vi "Stop Trigger Example.vi"() -> ()   [LabVIEW 2021]
uses:
  <vilib>/DAQmx/configure/timing.llb/DAQmx Timing (Sample Clock).vi
  <vilib>/DAQmx/configure/trigger.llb/DAQmx Reference Trigger (Digital Edge).vi
  <vilib>/DAQmx/create/channels.llb/DAQmx Create Channel (AI-Voltage-Basic).vi
  <vilib>/Utility/error.llb/DialogType.ctl
  <resource>/objmgr/daqmx.rc
  <vilib>/DAQmx/read.llb/DAQmx Read (Analog 1D Wfm NChan NSamp).vi
  <vilib>/DAQmx/configure/trigger.llb/DAQmx Start Trigger (Digital Edge).vi
panel:
  in  "Physical Channel(s)":tag="Dev1/ai0" caption="Physical Channel"
  in  "Sample Rate 2":dbl=10000.0 caption="Rate (Hz)" format="%0.2f"
  in  "Minimum Value":dbl=-10.0 format="%0.2f"
  in  "Maximum Value":dbl=10.0 format="%0.2f"
  in  "Stop Trigger Source":tag="/Dev1/PFI0"
  in  "Buffer Size 2":u32=100000
  out "data":waveform(dbl)[](array[waveform])
  in  "Start Trigger Source":tag="/Dev1/PFI1"
  in  "Post-Trigger Samples":u32
  in  "Samples Per Read":u32=100
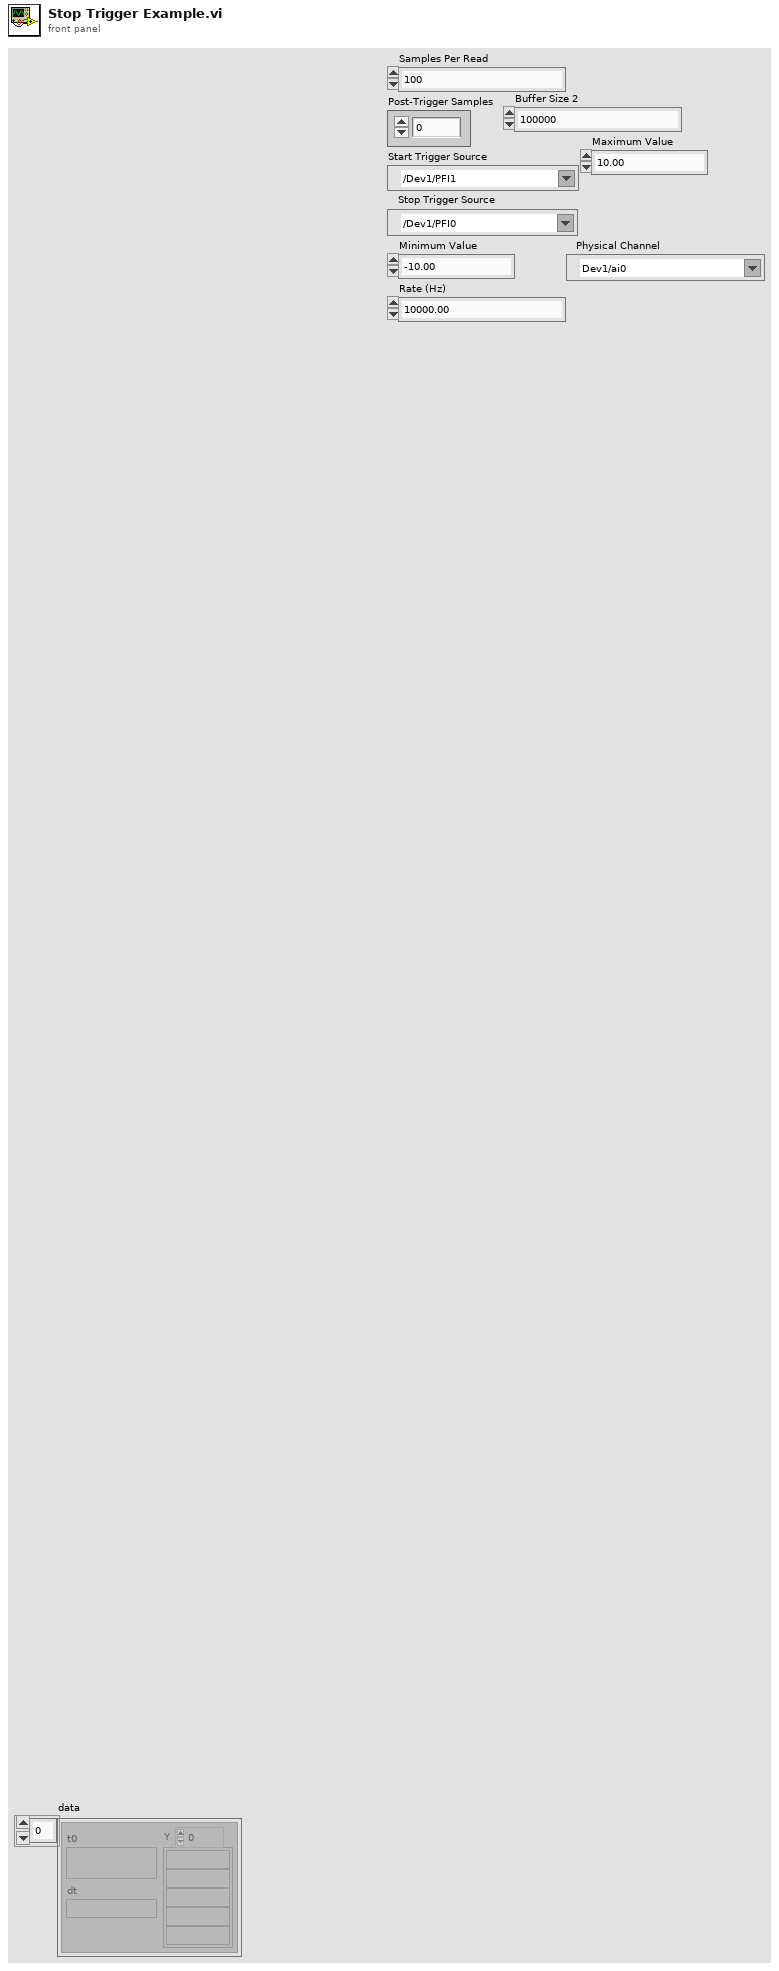
[diagram p1: front panel]
types:
  T1 = typedef "DialogType.ctl" = u16
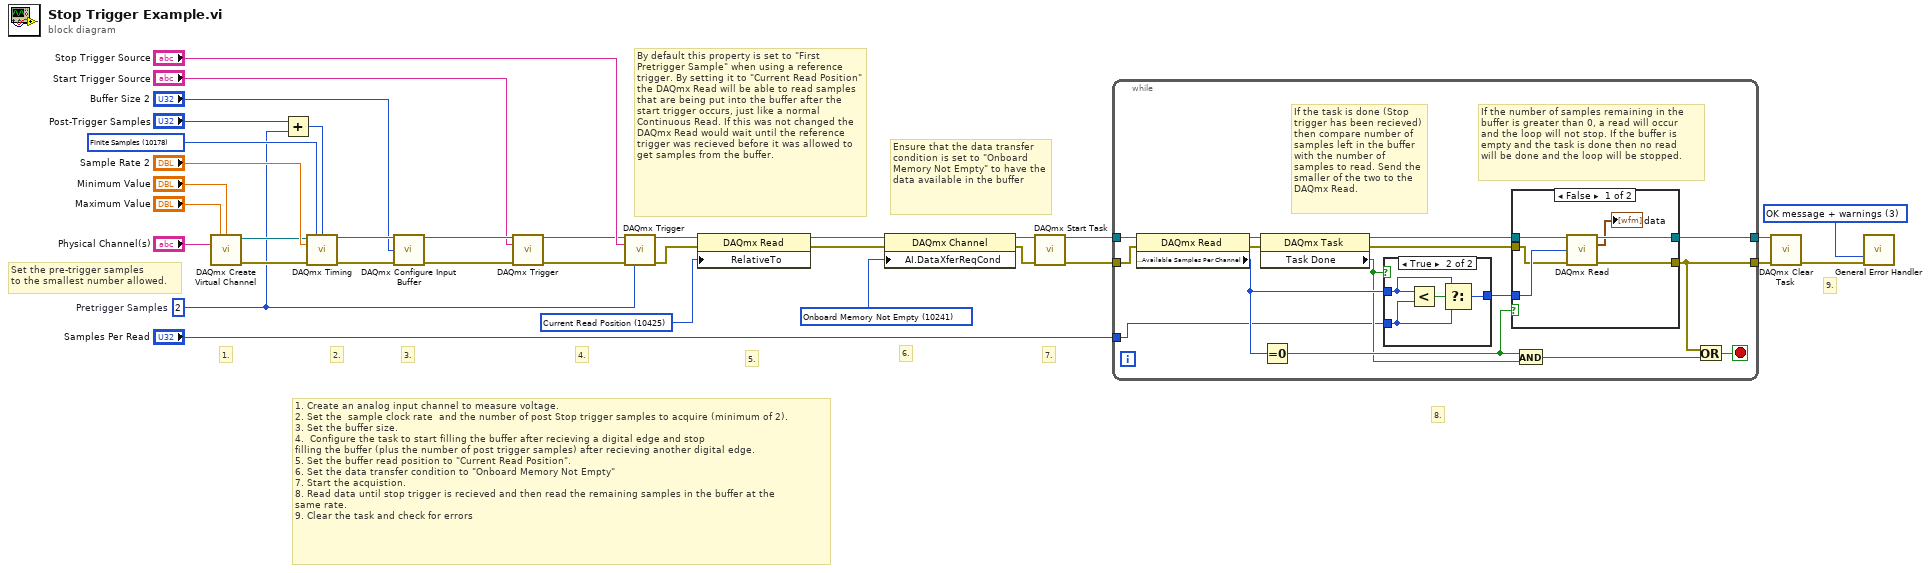
[diagram p0: block diagram]
diagram:
  w3 = 10241 items=["Onboard Memory More than Half Full"=10237, "Onboard Memory Not Empty"=10241, "Onboard Memory Custom Threshold"=12577, "When Acquisition Complete"=12546] ("AI.DataXferReqCond")
  w18 = 10425 items=["First Sample"=10424, "Current Read Position"=10425, "Reference Trigger"=10426, "First Pretrigger Sample"=10427, "Most Recent Sample"=10428] ("RelativeTo")
  w8 = u32 2  # Pretrigger Samples
  w24 = T1 3 items=["no dialog", "OK message", "continue or stop message", "OK message + warnings", "continue/stop + warnings"] ("type of dialog (OK msg:1)")
  w26 = 10178 items=["Finite Samples"=10178, "Continuous Samples"=10123] ("sample mode")
  # "Ensure that the data transfer condition is set to \"Onboard Memory Not Empty\" to have the data available in the buffer"
  # "7."
  # "Set the pre-trigger samples\nto the smallest number allowed."
  # "9."
  # "8."
  # "6."
  # "By default this property is set to \"First Pretrigger Sample\" when using a reference trigger. By setting it to \"Current Read Position\" the DAQmx Read will be able to read samples that are being put into the buffer after the start trigger occurs, just like a normal Continuous Read. If this was not changed the DAQmx Read would wait until the reference trigger was recieved before it was allowed to get samples from the buffer."
  # "5."
  # "1. Create an analog input channel to measure voltage.\n2. Set the  sample clock rate  and the number of post Stop trigger samples to acquire (minimum of 2).\n3. Set the buffer size.\n4.  Configure the task to start filling the buffer after recieving a digital edge and stop \nfilling the buffer (plus the number of post trigger samples) after recieving another digital edge.\n5. Set the buffer read position to \"Current Read Position\".\n6. Set the data transfer condition to \"Onboard Memory Not Empty\"\n7. Start the acquistion.\n8. Read data until stop trigger is recieved and then read the remaining samples in the buffer at the \nsame rate.\n9. Clear the task and check for errors"
  # "4."
  # "3."
  # "2."
  # "1."
  n1 = call-poly <vilib>:"DAQmx Create Virtual Channel.vi"("maximum value"="Maximum Value", "minimum value"="Minimum Value", "physical channels"="Physical Channel(s)") -> ("task out"=w29:refnum<k21>, "error out"=w32:errorcluster)  [unwired: 11 in]
  n2 = Add(x="Post-Trigger Samples", y=w8) -> (x+y=w9:u32)
  n3 = call-poly <vilib>:"DAQmx Timing.vi"("task/channels in"=w29, "sample mode"=w26, "samples per channel"=w9, "rate"="Sample Rate 2", "error in"=w32) -> ("task out"=w23:refnum<k21>, "error out"=w22:errorcluster)  [unwired: 9 in]
  n4 = call <vilib>:"DAQmx Configure Input Buffer.vi"("task/channels in"=w23, "buffer size (in samples per channel)"="Buffer Size 2", "error in"=w22) -> ("task out"=w14:refnum<k21>, "error out"=w13:errorcluster)  [unwired: 11 in]
  n5 = call-poly <vilib>:"DAQmx Trigger.vi"("task/channels in"=w14, "source"="Start Trigger Source", "error in"=w13) -> ("task out"=w11:refnum<k21>, "error out"=w12:errorcluster)  [unwired: 11 in]
  n6 = call-poly <vilib>:"DAQmx Trigger.vi"("task/channels in"=w11, "source"="Stop Trigger Source", "error in"=w12, "pretrigger samples per channel"=w8) -> ("task out"=w20:refnum<k21>, "error out"=w19:errorcluster)  [unwired: 10 in]
  n7 = property class="DAQmx Read"(reference=w20, error in=w19, "RelativeTo"=w18) -> (reference out=w5:refnum<k21>, error out=w4:errorcluster)
  n8 = property class="DAQmx Channel"(reference=w5, error in=w4, "AI.DataXferReqCond"=w3) -> (reference out=w2:refnum<k21>, error out=w1:errorcluster)
  n9 = call <vilib>:"DAQmx Start Task.vi"("task/channels in"=w2, "error in"=w1) -> ("task out"=w28:refnum<k21>, "error out"=w31:errorcluster)  [unwired: 12 in]
  n10 = while {
    tunnel: w31 -> [w47]
    tunnel: [w36] -> w15
    tunnel: w28 -> [w48]
    tunnel: [w46] -> w27
    tunnel: "Samples Per Read" -> [w35]
    stop <- w49 stop-if-true
    # "If the number of samples remaining in the\nbuffer is greater than 0, a read will occur\nand the loop will not stop. If the buffer is \nempty and the task is done then no read \nwill be done and the loop will be stopped."
    # "If the task is done (Stop trigger has been recieved) then compare number of samples left in the buffer\nwith the number of samples to read. Send the smaller of the two to the DAQmx Read."
    n11 = property class="DAQmx Read"(reference=w48, error in=w47) -> (reference out=w44:refnum<k21>, error out=w43:errorcluster, "Status:Available Samples Per Channel"=w45:u32)
    n12 = property class="DAQmx Task"(reference=w44, error in=w43) -> (reference out=w40:refnum<k21>, error out=w41:errorcluster, "Task Done"=w38:bool)
    n13 = Equal To 0?(x=w45) -> (x = 0?=w39:bool)
    n14 = case shown="True" w38 {
      tunnel: w45 -> [_ w61]
      tunnel: w35 -> [w58 w60]
      tunnel: [w58 w59] -> w42
      frame False {
      }
      frame True {
        n15 = Less?(x=w61, y=w60) -> (x < y?=w62:bool)
        n16 = Select(t=w61, s=w62, f=w60) -> (s? t:f=w59:u32)
      }
    }
    n17 = case shown="False" w39 {
      tunnel: [w55 w57] -> w36
      tunnel: [w54 w56] -> w46
      tunnel: w42 -> [w53 _]
      tunnel: w41 -> [w52 w57]
      tunnel: w40 -> [w51 w56]
      frame False {
        n18 = call-poly <vilib>:"DAQmx Read.vi"("task/channels in"=w51, "number of samples per channel"=w53, "error in"=w52) -> ("task out"=w54:refnum<k21>, "data"=→"data":waveform(dbl)[], "error out"=w55:errorcluster)  [unwired: 10 in]
      }
      frame True {
      }
    }
    n19 = And(x=w39, y=w38) -> (x .and. y?=w37:bool)
    n20 = Or(x=w36, y=w37) -> (x .or. y?=w49:bool)
  }
  n21 = call <vilib>:"DAQmx Clear Task.vi"("task in"=w27, "error in"=w15) -> ("error out"=w17:errorcluster)  [unwired: 13 in]
  n22 = call <vilib>:"General Error Handler.vi"("type of dialog (OK msg:1)"=w24, "error in (no error)"=w17) -> ()  [unwired: 9 in, 5 out]
